vi "build vector.vi"(9 "Index":i32, 10 "first element":dbl[][](array[numeric]), 11 "diff data":dbl[][](array[numeric])) -> (3 "Rebuild Vector":dbl[](array[numeric]))   [LabVIEW 2019]
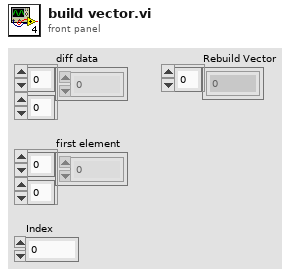
[diagram p1: front panel]
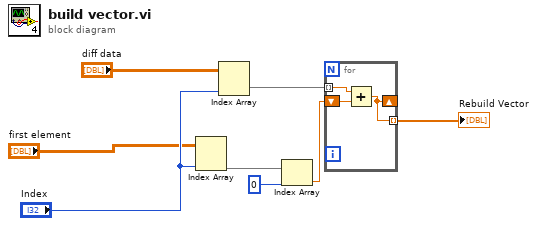
[diagram p0: block diagram]
diagram:
  n1 = Index Array(array="first element", index (col)="Index") -> (element=w3:dbl[])  [unwired: 1 in]
  n2 = Index Array(array="diff data", index (col)="Index") -> (element=w6:dbl[])  [unwired: 1 in]
  n3 = Index Array(array=w3, index=0) -> (element=w5:dbl)
  n4 = for {
    shift-right: [w9] -> _
    shift-left: w5 -> [w11]
    tunnel: w6 -> [w10] mode=indexing
    tunnel: [w9] -> w8 mode=indexing
    n5 = Add(x=w10, y=w11) -> (x+y=w9:dbl)
  }
  "Rebuild Vector" <- w8
